vi "read_c_string_at_memory_address.vi"(8 "error in (no error)":errorcluster, 11 "memory_address":u64) -> (0 "error out":errorcluster, 2 "string":string, 3 "memory_address out":u64)   [LabVIEW 2020, in "toml_edit.lvlib"]
uses:
  toml_edit.lvlib
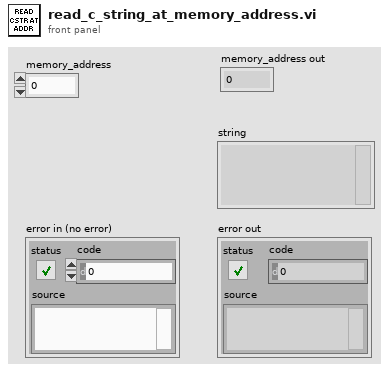
[diagram p1: front panel]
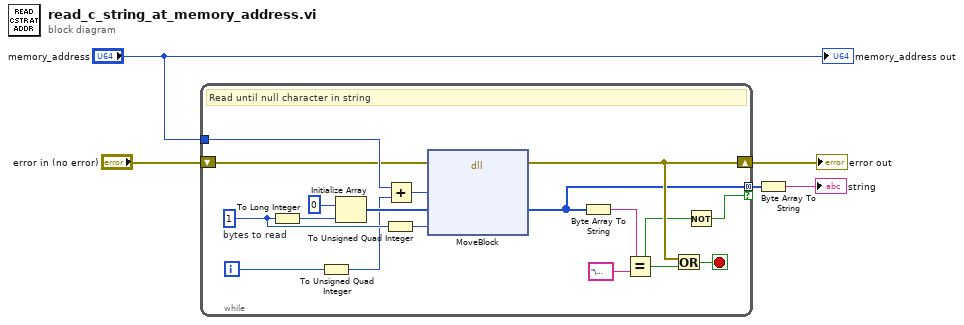
[diagram p0: block diagram]
diagram:
  n1 = while {
    tunnel: "memory_address" -> [w21]
    shift-right: [w9] -> w2
    shift-left: "error in (no error)" -> [w20]
    tunnel: [w7] -> w4 mode=concatenating if=w6
    i -> [w14]
    stop <- w10 stop-if-true
    w15 = u8 1  # bytes to read
    # "Read until null character in string"
    n2 = To Long Integer(number=w15) -> (32bit integer=w17:i32)
    n3 = To Unsigned Quad Integer(1:w14) -> (0:w11:u64)
    n4 = Initialize Array(u8 0, w17) -> (w18:u8[])
    n5 = To Unsigned Quad Integer(1:w15) -> (0:w16:u64)
    n6 = Add(x=w21, y=w11) -> (x+y=w22:u64)
    n7 = dll-call lib="LabVIEW" fn="MoveBlock"(error in=w20, "src"=w22, "dst"=w18, "size"=w16) -> (error out=w9:errorcluster, "dst"=w7:u8[])  [unwired: 5 in, 1 out]
    n8 = Byte Array To String(unsigned byte array=w7) -> (string=w12:string)
    n9 = Equal?(x=w12, y="\u0000" ("string")) -> (x = y?=w8:bool)
    n10 = Or(x=w9, y=w8) -> (x .or. y?=w10:bool)
    n11 = Not(x=w8) -> (.not. x?=w6:bool)
  }
  "error out" <- w2
  n12 = Byte Array To String(unsigned byte array=w4) -> (string=→"string":string)
  "memory_address out" <- "memory_address"
